vi "ep11_data_prog_control.vi"() -> ()   [LabVIEW 2019]
panel:
  out "Ans":dbl
  in  "Y":dbl
  in  "X":dbl
  in  "Enum":enum16{"Add", "Sub", "Mul", "Div"}(ring)
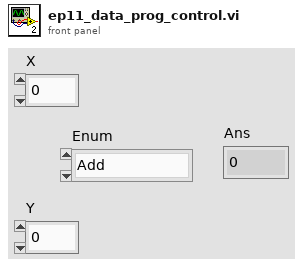
[diagram p1: front panel]
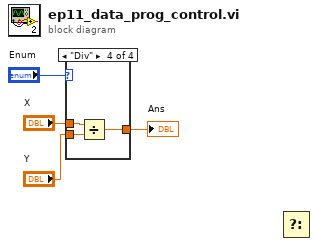
[diagram p0: block diagram]
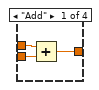
[diagram p2: hidden frame]
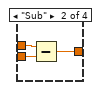
[diagram p3: hidden frame]
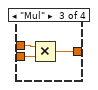
[diagram p4: hidden frame]
diagram:
  n1 = case shown="\"Div\"" "Enum" {
    tunnel: "X" -> [w7 w10 w13 w16]
    tunnel: "Y" -> [w6 w9 w12 w15]
    tunnel: [w5 w8 w11 w14] -> w1
    frame "Add" {
      n2 = Add(x=w7, y=w6) -> (x+y=w5:dbl)
    }
    frame "Sub" {
      n3 = Subtract(x=w10, y=w9) -> (x-y=w8:dbl)
    }
    frame "Mul" {
      n4 = Multiply(x=w13, y=w12) -> (x*y=w11:dbl)
    }
    frame "Div" {
      n5 = Divide(x=w16, y=w15) -> (x/y=w14:dbl)
    }
  }
  "Ans" <- w1
  n6 = Select() -> ()  [unwired: 3 in, 1 out]
